vi "Set Options to DVR.vi"(8 "Error In":errorcluster, 10 "Options":T1, 11 "Options DVR":T2) -> (0 "Error Out":errorcluster, 3 "Options DVR":T2)   [LabVIEW 2011]
uses:
  Controls/Options DVR.ctl
  Controls/Options.ctl
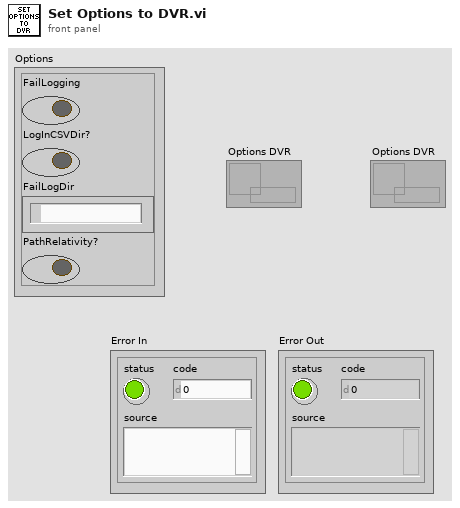
[diagram p1: front panel]
types:
  T1 = typedef "Options.ctl" = cluster{"FailLogging":bool, "LogInCSVDir?":bool, "FailLogDir":path, "PathRelativity?":bool}
  T2 = typedef "Options DVR.ctl" = refnum<data-value>
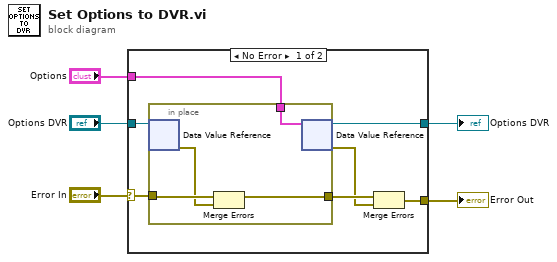
[diagram p0: block diagram]
diagram:
  n1 = case shown="No Error" "Error In" {
    selector: "Error In" -> [w7 w18]
    tunnel: "Options DVR" -> [w12 w17]
    tunnel: [w9 w18] -> w4
    tunnel: [w8 w17] -> w3
    tunnel: "Options" -> [w6 _]
    frame No Error {
      n2 = in-place {
        in-place-border: w7 -> [w16]
        in-place-border: [w14] -> w11
        in-place-border: w6 -> [w13]
        n3 = in-place-dvr #1(w12) -> (w15:errorcluster)  [unwired: 1 out]
        n4 = Merge Errors(w16, w15) -> (w14:errorcluster)
        n5 = in-place-dvr #1(w13) -> (w8:T2, w10:errorcluster)
      }
      n6 = Merge Errors(w11, w10) -> (w9:errorcluster)
    }
    frame Error {
    }
  }
  "Error Out" <- w4
  "Options DVR" <- w3
